vi "SMR_LabVIEW_V8.3.vi"() -> ()   [LabVIEW 2025]
uses:
  <vilib>/DAQmx/write.llb/DAQmx Write (Analog DBL 1Chan 1Samp).vi
  <vilib>/DAQmx/read.llb/DAQmx Read (Analog 1D DBL NChan 1Samp).vi
  <vilib>/DAQmx/read.llb/DAQmx Read (Analog 2D DBL NChan NSamp).vi
  <vilib>/Analysis/baseanly.llb/Mean (DBL).vi
  <vilib>/DAQmx/create/channels.llb/DAQmx Create Channel (AI-Temperature-Thermocouple).vi
  <vilib>/DAQmx/create/channels.llb/DAQmx Create Channel (AI-Voltage-Basic).vi
  <vilib>/DAQmx/create/channels.llb/DAQmx Create Channel (AO-Voltage-Basic).vi
  <vilib>/DAQmx/miscellaneous.llb/DAQmx Fill In Error Info.vi
  <vilib>/DAQmx/configure/timing.llb/DAQmx Timing (Sample Clock).vi
  <vilib>/addons/control/pid/pid.llb/PID (DBL).vi
  <vilib>/measure/maspectr.llb/FFT Power Spectrum and PSD for 1 Chan.vi
  <vilib>/measure/matone.llb/Extract Single Tone Information 1 Chan.vi
  <vilib>/addons/control/pid/NI_PID_pid.lvlib
  <vilib>/Analysis/NI_AALBase.lvlib
  <vilib>/ptbypt/NI_PtbyPt.lvlib
  <vilib>/measure/NI_MAPro.lvlib
panel:
  out "HW Valve Command (V)":dbl
  in  "HX Flow Setpoint (GPM)":dbl
  in  "Manual HW Valve Voltage (V)":dbl
  in  "HW Valve: Manual / PID":bool
  in  "PID gains for HW Valve":T1={"proportional gain (Kc)"=1.0, "integral time (Ti, min)"=0.01, "derivative time (Td, min)"=0.0} {"derivative time (Td, min)" format="%.3f"; "integral time (Ti, min)" format="%.3f"; "proportional gain (Kc)" format="%.3f"}
  out "Rod Power (W)":dbl
  out "Current Through Rod (A)":dbl
  out "Time in Steady State (s)":dbl
  in  "Steady-State Dwell (s)":dbl
  out "Main Loop Flow (GPM)":dbl
  out "FM Amplitude":dbl
  out "FM Frequency":dbl
  out "Spectrum":cluster{"f0":dbl, "df":dbl, "magnitude":dbl[]}(graph)
  out "Raw Signal":waveform(dbl)(graph)
  out "Smoothed HX Flow (GPM)":dbl
  out "Flow History":dbl(graph)
  out "HX Flow (GPM)":dbl
  out "Voltage Across Rod (V)":dbl format="%0.2f"
  out "Current Run Folder":path
  in  "Log Root Folder":path=path "C:/Users/LocalUser/Documents/GitHub/thermal-loop/resources/v0.1.1/data/001"
  out "Raw NI9201 \nVoltage Display":T2
  in  "Loop Period (ms)":dbl=1000.0
  in  "Stop":bool
  out "Auto Steady State Threshold (deg C/min)":dbl
  out "Max dT/dt (deg C/min)":dbl
  out "Temp Change Rate (deg C/min)":dbl
  out "5-Min Baseline Complete":bool
  out "Rate Window Ready":bool
  out "Steady State":bool
  in  "Voltage Limit (V)":dbl=10.0
  in  "Temperature Limit (C)":dbl=50.0
  in  "Pressure Limit (psi)":dbl=15.0
  out "Max Voltage":bool
  out "Max Temperature":bool
  out "Max Pressure":bool
  out "Heat Exchanger Pressure History":dbl(graph)
  out "Main Loop Pressure History":T3(graph)
  out "Overall Avg Pressure (psi)":dbl
  out "Heat Exchanger Pressure P6 (psi)":dbl
  out "Main Loop Avg Pressure (psi)":dbl
  out "Pressure Display":T4
  out "Overall Pressure History":T5(graph)
  out "Max Loop Pressure (psi)":dbl
  out "Heat Exchanger Temperature History":cluster{"Waveform":dbl, "Waveform":dbl}(graph)
  out "Main Loop Temeperature History":T6(graph)
  out "Heat Exchanger Avg Temp (deg C)":dbl
  out "Temperature Display":T7
  out "Overall Temperature History":T8(graph)
  out "Overall Avg Temp (deg C)":dbl
  out "Max Loop Temp (deg C)":dbl
  out "Final P-Valve Voltage (V)":dbl
  out "PID Trim Voltage (V)":dbl
  in  "PID Temp Setpoint (deg C)":dbl
  in  "Auto PID Enable":bool
  in  "Manual P-Valve Voltage (V)":dbl min=0.0 max=10.0
  out "Main Loop Avg Temp (deg C)":dbl
  # "HoneyWell Valve Control"
  # "Heat Exchanger Flow"
  # "Control/Troubleshoot"
  # "Steady State"
  # "Emergency Indicators"
  # "Pressure"
  # "Temperature"
  # "Proportional Valve Control"
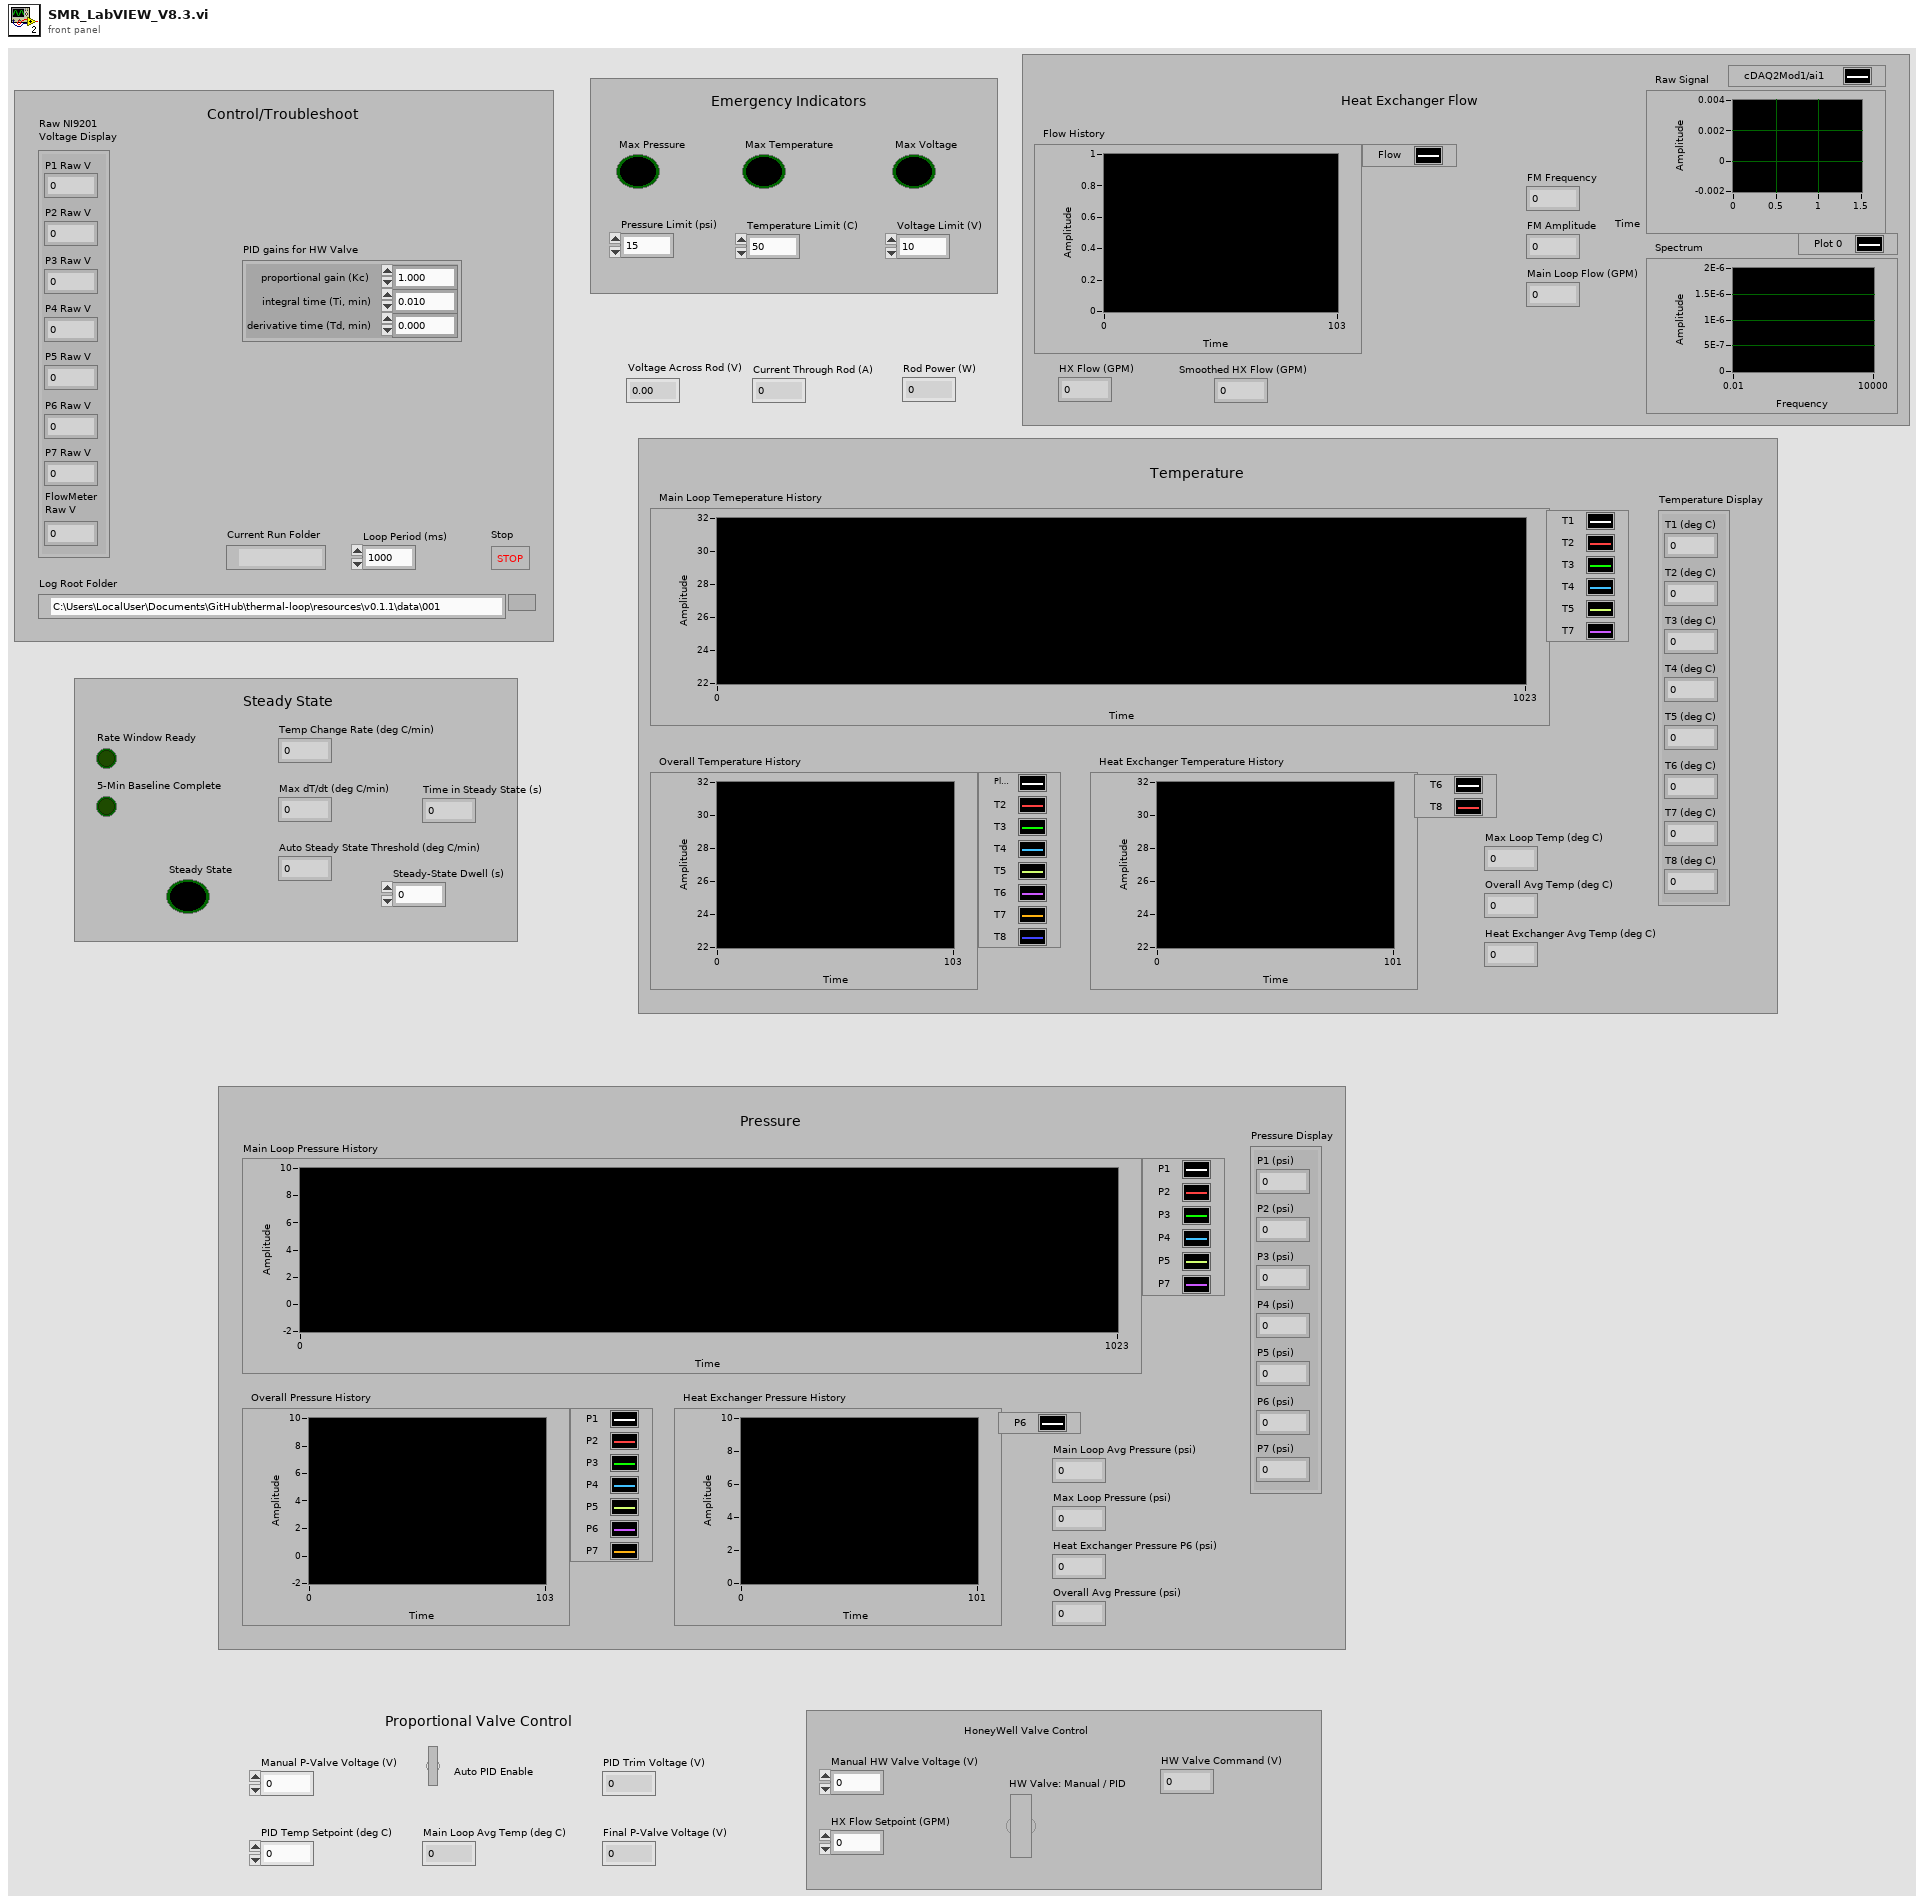
[diagram p1: front panel]
types:
  T1 = cluster{"proportional gain (Kc)":dbl, "integral time (Ti, min)":dbl, "derivative time (Td, min)":dbl}
  T2 = cluster{"P1 Raw V":dbl, "P2 Raw V":dbl, "P3 Raw V":dbl, "P4 Raw V":dbl, "P5 Raw V":dbl, "P6 Raw V":dbl, "P7 Raw V":dbl, "FlowMeter\nRaw V":dbl}
  T3 = cluster{"P1":dbl, "P2":dbl, "P3":dbl, "P4":dbl, "P5":dbl, "P7":dbl}
  T4 = cluster{"P1 (psi)":dbl, "P2 (psi)":dbl, "P3 (psi)":dbl, "P4 (psi)":dbl, "P5 (psi)":dbl, "P6 (psi)":dbl, "P7 (psi)":dbl}
  T5 = cluster{"P1":dbl, "P2":dbl, "P3":dbl, "P4":dbl, "P5":dbl, "P6":dbl, "P7":dbl}
  T6 = cluster{"Waveform":dbl, "Waveform":dbl, "Waveform":dbl, "Waveform":dbl, "Waveform":dbl, "Waveform":dbl}
  T7 = cluster{"T1 (deg C)":dbl, "T2 (deg C)":dbl, "T3 (deg C)":dbl, "T4 (deg C)":dbl, "T5 (deg C)":dbl, "T6 (deg C)":dbl, "T7 (deg C)":dbl, "T8 (deg C)":dbl}
  T8 = cluster{"Waveform":dbl, "Waveform":dbl, "Waveform":dbl, "Waveform":dbl, "Waveform":dbl, "Waveform":dbl, "Waveform":dbl, "Waveform":dbl}
  T9 = enum16{"open", "replace", "create", "open or create", "replace or create", "replace or create with confirmation"}
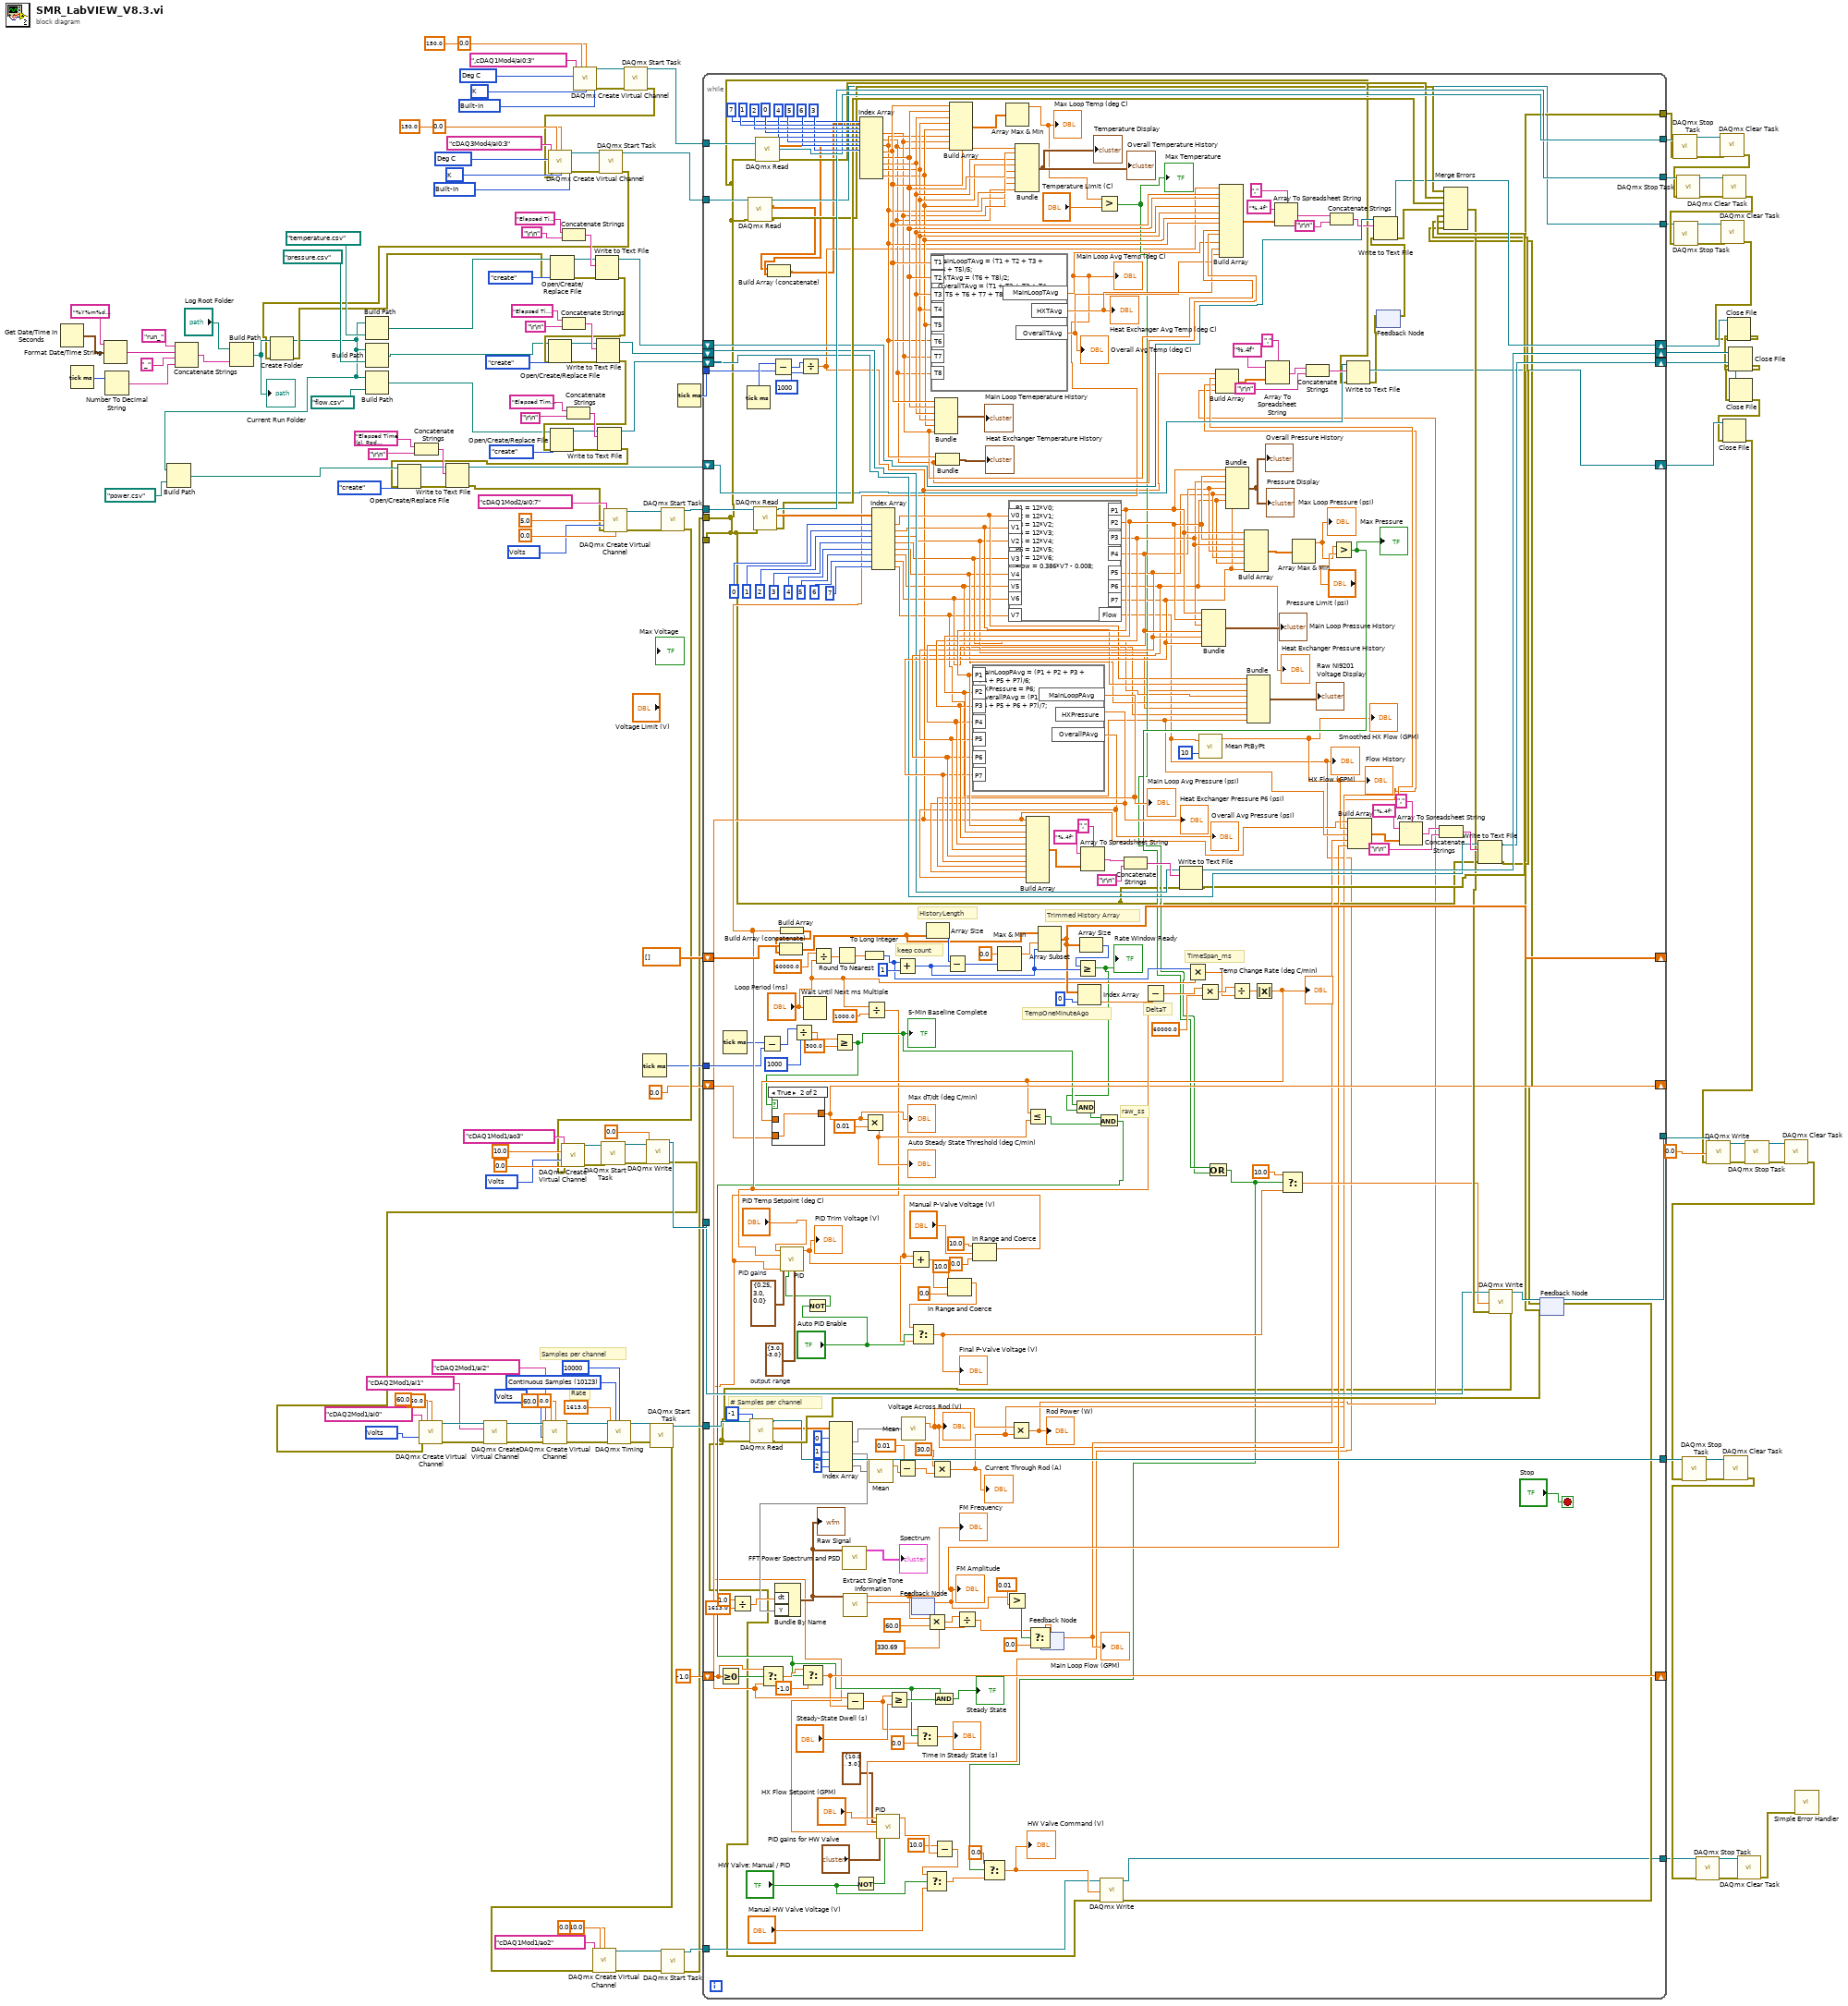
[diagram p0: block diagram]
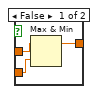
[diagram p2: hidden frame]
diagram:
  w17 = 10348 items=["Volts"=10348, "From Custom Scale"=10065] ("units")
  w34 = 10200 items=["Built-In"=10200, "Constant Value"=10116, "Channel"=10113] ("cjc source")
  w35 = 10073 items=["J"=10072, "K"=10073, "N"=10077, "R"=10082, "S"=10085, "T"=10086, "B"=10047, "E"=10055] ("thermocouple type")
  w36 = 10143 items=["Deg C"=10143, "Deg F"=10144, "Kelvins"=10325, "Deg R"=10145, "From Custom Scale"=10065] ("units")
  w66 = 10123 items=["Finite Samples"=10178, "Continuous Samples"=10123, "Hardware Timed Single Point"=12522] ("sample mode")
  w68 = 10348 items=["Volts"=10348, "From Custom Scale"=10065] ("units")
  w87 = 10348 items=["Volts"=10348, "From Custom Scale"=10065] ("units")
  w149 = 10200 items=["Built-In"=10200, "Constant Value"=10116, "Channel"=10113] ("cjc source")
  w150 = 10073 items=["J"=10072, "K"=10073, "N"=10077, "R"=10082, "S"=10085, "T"=10086, "B"=10047, "E"=10055] ("thermocouple type")
  w151 = 10143 items=["Deg C"=10143, "Deg F"=10144, "Kelvins"=10325, "Deg R"=10145, "From Custom Scale"=10065] ("units")
  w158 = 10348 items=["Volts"=10348, "From Custom Scale"=10065] ("units")
  # "Samples per channel"
  # "Rate"
  n1 = Get Date/Time In Seconds() -> (seconds since 1Jan1904=w108:timestamp)
  n2 = Tick Count (ms)() -> (millisecond timer value=w106:u32)
  n3 = Format Date/Time String(time format string (%c)="%Y%m%d_%H%M%S", seconds (now)=w108) -> (date/time string=w103:string)  [unwired: 1 in]
  n4 = Number To Decimal String(number=w106) -> (decimal integer string=w104:string)  [unwired: 1 in]
  n5 = Concatenate Strings("run_" ("string"), w103, "_" ("string"), w104) -> (w100:string)
  n6 = Build Path(base path="Log Root Folder", name or relative path=w100) -> (appended path=w99:path)
  "Current Run Folder" <- w99
  n7 = Concatenate Strings("Elapsed Time (s), Rod voltage (V), Rod Current (A), Rod Power (W)", "\r\n") -> (w53:string)
  n8 = Concatenate Strings("Elapsed Time (s),T1 (deg C),T2 (deg C),T3 (deg C),T4 (deg C),T5 (deg C),T6 (deg C),T7 (deg C),T8 (deg C),Main Loop Avg Temp (deg C),HX Avg Temp (deg C),Overall Avg Temp (deg C)", "\r\n") -> (w132:string)
  n9 = Concatenate Strings("Elapsed Time (s),P1 (psi),P2 (psi),P3 (psi),P4 (psi),P5 (psi),P6 (psi),P7 (psi),Main Loop Avg Pressure (psi),HX Pressure (psi),Overall Avg Pressure (psi)", "\r\n") -> (w130:string)
  n10 = Concatenate Strings("Elapsed Time (s),Heat Exchanger Flow (GPM),Flow Raw Voltage (V), Main Loop Flow (GPM), Flow Signal Amplitude (V)", "\r\n") -> (w126:string)
  n11 = call-poly <vilib>:"DAQmx Create Virtual Channel.vi"("maximum value"=150.0, "minimum value"=0.0, "physical channels"=tag ",cDAQ1Mod4/ai0:3", "cjc source"=w149, "units"=w151, "thermocouple type"=w150) -> ("task out"=w148:refnum<k21>, "error out"=w147:errorcluster)  [unwired: 8 in]
  n12 = call <vilib>:"DAQmx Start Task.vi"("task/channels in"=w148, "error in"=w147) -> ("task out"=w146:refnum<k21>, "error out"=w30:errorcluster)  [unwired: 12 in]
  n13 = call-poly <vilib>:"DAQmx Create Virtual Channel.vi"("maximum value"=150.0, "minimum value"=0.0, "physical channels"=tag "cDAQ3Mod4/ai0:3", "cjc source"=w34, "units"=w36, "error in"=w30, "thermocouple type"=w35) -> ("task out"=w33:refnum<k21>, "error out"=w32:errorcluster)  [unwired: 7 in]
  n14 = call <vilib>:"DAQmx Start Task.vi"("task/channels in"=w33, "error in"=w32) -> ("task out"=w28:refnum<k21>, "error out"=w29:errorcluster)  [unwired: 12 in]
  n15 = Create Folder(path (use dialog)=w99, error in=w29) -> (created path=w47:path, error out=w92:errorcluster)  [unwired: 1 in, 1 out]
  n16 = Build Path(base path=w47, name or relative path=path "power.csv") -> (appended path=w48:path)
  n17 = Build Path(base path=w47, name or relative path=path "temperature.csv") -> (appended path=w98:path)
  n18 = Build Path(base path=w47, name or relative path=path "pressure.csv") -> (appended path=w97:path)
  n19 = Build Path(base path=w47, name or relative path=path "flow.csv") -> (appended path=w96:path)
  n20 = Open/Create/Replace File(file path (use dialog)=w98, error in=w92, operation (0:open)=T9."create") -> (refnum out=w131:refnum<file>, error out=w115:errorcluster)  [unwired: 3 in, 1 out]
  n21 = Write to Text File(file (use dialog)=w131, text=w132, error in=w115) -> (refnum out=w122:refnum<file>, error out=w114:errorcluster)  [unwired: 1 in, 1 out]
  n22 = Open/Create/Replace File(file path (use dialog)=w97, error in=w114, operation (0:open)=T9."create") -> (refnum out=w129:refnum<file>, error out=w113:errorcluster)  [unwired: 3 in, 1 out]
  n23 = Write to Text File(file (use dialog)=w129, text=w130, error in=w113) -> (refnum out=w121:refnum<file>, error out=w112:errorcluster)  [unwired: 1 in, 1 out]
  n24 = Open/Create/Replace File(file path (use dialog)=w96, error in=w112, operation (0:open)=T9."create") -> (refnum out=w125:refnum<file>, error out=w111:errorcluster)  [unwired: 3 in, 1 out]
  n25 = Write to Text File(file (use dialog)=w125, text=w126, error in=w111) -> (refnum out=w120:refnum<file>, error out=w45:errorcluster)  [unwired: 1 in, 1 out]
  n26 = Open/Create/Replace File(file path (use dialog)=w48, error in=w45, operation (0:open)=T9."create") -> (refnum out=w52:refnum<file>, error out=w49:errorcluster)  [unwired: 3 in, 1 out]
  n27 = Write to Text File(file (use dialog)=w52, text=w53, error in=w49) -> (refnum out=w43:refnum<file>, error out=w44:errorcluster)  [unwired: 1 in, 1 out]
  n28 = call-poly <vilib>:"DAQmx Create Virtual Channel.vi"("maximum value"=5.0, "minimum value"=0.0, "physical channels"=tag "cDAQ1Mod2/ai0:7", "units"=w158, "error in"=w44) -> ("task out"=w157:refnum<k21>, "error out"=w156:errorcluster)  [unwired: 9 in]
  n29 = Tick Count (ms)() -> (millisecond timer value=w73:u32)
  n30 = call <vilib>:"DAQmx Start Task.vi"("task/channels in"=w157, "error in"=w156) -> ("task out"=w155:refnum<k21>, "error out"=w80:errorcluster)  [unwired: 12 in]
  n31 = call-poly <vilib>:"DAQmx Create Virtual Channel.vi"("maximum value"=10.0, "minimum value"=0.0, "physical channels"=tag "cDAQ1Mod1/ao3", "units"=w87, "error in"=w80) -> ("task out"=w86:refnum<k21>, "error out"=w85:errorcluster)  [unwired: 9 in]
  n32 = call <vilib>:"DAQmx Start Task.vi"("task/channels in"=w86, "error in"=w85) -> ("task out"=w84:refnum<k21>, "error out"=w83:errorcluster)  [unwired: 12 in]
  n33 = call-poly <vilib>:"DAQmx Write.vi"("task/channels in"=w84, "data"=0.0, "error in"=w83) -> ("task out"=w81:refnum<k21>, "error out"=w60:errorcluster)  [unwired: 10 in, 1 out]
  n34 = call-poly <vilib>:"DAQmx Create Virtual Channel.vi"("maximum value"=60.0, "minimum value"=-60.0, "physical channels"=tag "cDAQ2Mod1/ai0", "units"=w68, "error in"=w60) -> ("task out"=w57:refnum<k21>, "error out"=w56:errorcluster)  [unwired: 9 in]
  n35 = call-poly <vilib>:"DAQmx Create Virtual Channel.vi"("task in"=w57, "physical channels"=tag "cDAQ2Mod1/ai1", "error in"=w56) -> ("task out"=w21:refnum<k21>, "error out"=w19:errorcluster)  [unwired: 11 in]
  n36 = call-poly <vilib>:"DAQmx Create Virtual Channel.vi"("task in"=w21, "maximum value"=60.0, "minimum value"=-60.0, "physical channels"=tag "cDAQ2Mod1/ai2", "units"=w17, "error in"=w19) -> ("task out"=w20:refnum<k21>, "error out"=w18:errorcluster)  [unwired: 8 in]
  n37 = call-poly <vilib>:"DAQmx Timing.vi"("task/channels in"=w20, "sample mode"=w66, "samples per channel"=10000, "rate"=1613.0, "error in"=w18) -> ("task out"=w64:refnum<k21>, "error out"=w63:errorcluster)  [unwired: 9 in]
  n38 = call <vilib>:"DAQmx Start Task.vi"("task/channels in"=w64, "error in"=w63) -> ("task out"=w59:refnum<k21>, "error out"=w8:errorcluster)  [unwired: 12 in]
  n39 = call-poly <vilib>:"DAQmx Create Virtual Channel.vi"("maximum value"=10.0, "minimum value"=0.0, "physical channels"=tag "cDAQ1Mod1/ao2", "error in"=w8) -> ("task out"=w11:refnum<k21>, "error out"=w10:errorcluster)  [unwired: 10 in]
  n40 = call <vilib>:"DAQmx Start Task.vi"("task/channels in"=w11, "error in"=w10) -> ("task out"=w9:refnum<k21>, "error out"=w7:errorcluster)  [unwired: 12 in]
  n41 = Tick Count (ms)() -> (millisecond timer value=w119:u32)
  n42 = while {
    tunnel: w155 -> [w403]
    tunnel: w146 -> [w386]
    tunnel: [w377] -> w145
    tunnel: [w196] -> _
    tunnel: [w376] -> w144
    tunnel: [w255] -> w143
    shift-right: [w353] -> w118
    shift-left: w122 -> [w354]
    shift-right: [w334] -> w117
    shift-left: w121 -> [w335]
    shift-right: [w326] -> w116
    shift-left: w120 -> [w327]
    tunnel: w119 -> [w372]
    shift-right: [w305] -> _
    shift-left: dbl[] [] -> [w318]
    tunnel: w81 -> [w287]
    tunnel: w7 -> [w196]
    tunnel: [w293] -> w78
    tunnel: w73 -> [w276]
    shift-right: [w269] -> _
    shift-left: 0.0 -> [w271]
    tunnel: w59 -> [w254]
    tunnel: [w253] -> w58
    shift-right: [w213] -> w42
    shift-left: w43 -> [w214]
    shift-right: [w205] -> _
    shift-left: -1.0 -> [w209]
    tunnel: w28 -> [w197]
    tunnel: [w194] -> w24
    tunnel: w9 -> [w167]
    tunnel: [w163] -> w2
    stop <- "Stop" stop-if-true
    w291 = cluster{"output high":dbl, "output low":dbl} {"output high"=3.0, "output low"=-3.0}  # output range
    w292 = T1 {"proportional gain (Kc)"=0.25, "integral time (Ti, min)"=3.0, "derivative time (Td, min)"=0.0}  # PID gains
    # "raw_ss"
    # "# Samples per channel"
    # "TimeSpan_ms"
    # "DeltaT"
    # "TempOneMinuteAgo"
    # "Trimmed History Array"
    # "HistoryLength"
    # "keep count"
    n43 = Greater Or Equal To 0?(x=w209) -> (x >= 0?=w210:bool)
    n44 = Tick Count (ms)() -> (millisecond timer value=w277:u32)
    n45 = Divide(x=1.0, y=1613.0) -> (x/y=w227:dbl)
    n46 = Tick Count (ms)() -> (millisecond timer value=w373:u32)
    n47 = call-poly <vilib>:"DAQmx Read.vi"("task/channels in"=w197, "error in"=w196) -> ("task out"=w194:refnum<k21>, "data"=w191:dbl[], "error out"=w195:errorcluster)  [unwired: 11 in]
    n48 = call-poly <vilib>:"DAQmx Read.vi"("task/channels in"=w403, "error in"=w196) -> ("task out"=w376:refnum<k21>, "data"=w394:dbl[], "error out"=w374:errorcluster)  [unwired: 11 in]
    n49 = call-poly <vilib>:"DAQmx Read.vi"("task/channels in"=w386, "error in"=w196) -> ("task out"=w377:refnum<k21>, "data"=w192:dbl[], "error out"=w375:errorcluster)  [unwired: 11 in]
    n50 = Subtract(x=w277, y=w276) -> (x-y=w275:u32)
    n51 = Build Array (concatenate)(w191, w192) -> (w193:dbl[])
    n52 = Subtract(x=w373, y=w372) -> (x-y=w371:u32)
    n53 = Divide(x=w275, y=u32 1000) -> (x/y=w273:dbl)
    n54 = Divide(x=w371, y=u32 1000) -> (x/y=w206:dbl)
    n55 = Select(t=w209, s=w210, f=w206) -> (s? t:f=w208:dbl)
    n56 = Wait Until Next ms Multiple(millisecond multiple="Loop Period (ms)") -> ()  [unwired: 1 out]
    n57 = Not(x="Auto PID Enable") -> (.not. x?=w288:bool)
    n58 = Divide(x=60000.0, y="Loop Period (ms)") -> (x/y=w315:dbl)
    n59 = Greater Or Equal?(x=w273, y=300.0) -> (x >= y?=w266:bool)
    "5-Min Baseline Complete" <- w266
    n60 = Round To Nearest(number=w315) -> (nearest integer value=w314:dbl)
    n61 = Not(x="HW Valve: Manual / PID") -> (.not. x?=w177:bool)
    n62 = Index Array(array=w193, index #1=7 ("index"), index #2=1 ("index"), index #3=2 ("index"), index #4=0 ("index"), index #5=4 ("index"), index #6=5 ("index"), index #7=6 ("index"), index #8=3 ("index")) -> (element #1=w363:dbl, element #2=w362:dbl, element #3=w364:dbl, element #4=w369:dbl, element #5=w368:dbl, element #6=w367:dbl, element #7=w366:dbl, element #8=w365:dbl)
    n63 = To Long Integer(number=w314) -> (32bit integer=w302:i32)
    n64 = Divide(x="Loop Period (ms)", y=1000.0) -> (x/y=w162:dbl)
    n65 = Index Array(array=w394, index #1=0 ("index"), index #2=1 ("index"), index #3=2 ("index"), index #4=3 ("index"), index #5=4 ("index"), index #6=5 ("index"), index #7=6 ("index"), index #8=7 ("index")) -> (element #1=w252:dbl, element #2=w251:dbl, element #3=w250:dbl, element #4=w249:dbl, element #5=w248:dbl, element #6=w247:dbl, element #7=w246:dbl, element #8=w245:dbl)
    n66 = Add(x=w302, y=1) -> (x+y=w307:i32)
    n67 = feedback #1() -> (w223:dbl)  [unwired: 1 in]
    "FM Amplitude" <- w223
    n68 = formula code="MainLoopTAvg = (T1 + T2 + T3 + T4 + T5)/5;\nHXTAvg = (T6 + T8)/2;\nOverallTAvg = (T1 + T2 + T3 + T4 + T5 + T6 + T7 + T8)/8;"("T1"=w369, "T2"=w368, "T3"=w367, "T4"=w366, "T5"=w365, "T6"=w364, "T7"=w363, "T8"=w362) -> ("MainLoopTAvg"=w279:dbl, "HXTAvg"=w361:dbl, "OverallTAvg"=w360:dbl)
    "Overall Avg Temp (deg C)" <- w360
    "Main Loop Avg Temp (deg C)" <- w279
    "Heat Exchanger Avg Temp (deg C)" <- w361
    n69 = Build Array(w279) -> (w317:dbl[])
    n70 = Build Array (concatenate)(w318, w317) -> (w309:dbl[])
    n71 = call-poly <vilib>:"PID.vi"("reinitialize? (F)"=w288, "output range"=w291, "dt (s)"=w162, "PID gains"=w292, "process variable"=w279, "setpoint"="PID Temp Setpoint (deg C)") -> ("output"=w286:dbl)  [unwired: 4 in, 1 out]
    "PID Trim Voltage (V)" <- w286
    n72 = Array Size(array=w309) -> (size(s)=w312:i32)
    n73 = Bundle("Waveform"=w369, "Waveform"=w368, "Waveform"=w367, "Waveform"=w366, "Waveform"=w365, "Waveform"=w363) -> (→"Main Loop Temeperature History":T6)  [unwired: 1 in]
    n74 = Bundle("Waveform"=w364, "Waveform"=w362) -> (→"Heat Exchanger Temperature History":cluster{"Waveform":dbl, "Waveform":dbl})  [unwired: 1 in]
    n75 = Subtract(x=w312, y=w307) -> (x-y=w310:i32)
    n76 = Build Array(w369, w368, w367, w366, w365, w364, w363, w362) -> (w404:dbl[])
    n77 = In Range and Coerce(upper limit=10.0, x="Manual P-Valve Voltage (V)", lower limit=0.0) -> (coerced(x)=w281:dbl)  [unwired: 1 out]
    n78 = Add(x=w281, y=w286) -> (x+y=w285:dbl)
    n79 = In Range and Coerce(upper limit=10.0, x=w285, lower limit=0.0) -> (coerced(x)=w280:dbl)  [unwired: 1 out]
    n80 = Select(t=w280, s="Auto PID Enable", f=w281) -> (s? t:f=w258:dbl)
    "Final P-Valve Voltage (V)" <- w258
    n81 = Max & Min(x=0.0, y=w310) -> (max(x,y)=w308:dbl)  [unwired: 1 out]
    n82 = Array Max & Min(array=w404) -> (max value=w320:dbl)  [unwired: 3 out]
    "Max Loop Temp (deg C)" <- w320
    n83 = Greater?(x=w223, y=0.01) -> (0:w231:bool)
    n84 = formula code="P1 = 12*V0;\nP2 = 12*V1;\nP3 = 12*V2;\nP4 = 12*V3;\nP5 = 12*V4;\nP6 = 12*V5; \nP7 = 12*V6;\nFlow = 0.386*V7 - 0.008;"("V0"=w252, "V1"=w251, "V2"=w250, "V3"=w249, "V4"=w248, "V5"=w247, "V6"=w246, "V7"=w245) -> ("P1"=w352:dbl, "P2"=w351:dbl, "P3"=w350:dbl, "P4"=w349:dbl, "P5"=w348:dbl, "P6"=w347:dbl, "P7"=w346:dbl, "Flow"=w180:dbl)
    "HX Flow (GPM)" <- w180
    "Heat Exchanger Pressure History" <- w347
    n85 = call-poly <vilib>:"PID.vi"("reinitialize? (F)"=w177, "output range"=cluster{"output high":dbl, "output low":dbl} {"output high"=10.0, "output low"=3.0}, "dt (s)"=w162, "PID gains"="PID gains for HW Valve", "process variable"=w180, "setpoint"="HX Flow Setpoint (GPM)") -> ("output"=w176:dbl)  [unwired: 4 in, 1 out]
    n86 = Subtract(x=10.0, y=w176) -> (x-y=w173:dbl)
    n87 = Select(t=w173, s="HW Valve: Manual / PID", f="Manual HW Valve Voltage (V)") -> (s? t:f=w170:dbl)
    n88 = formula code="MainLoopPAvg = (P1 + P2 + P3 + P4 + P5 + P7)/6;\nHXPressure = P6;\nOverallPAvg = (P1 + P2 + P3 + P4 + P5 + P6 + P7)/7;"("P1"=w352, "P2"=w351, "P3"=w350, "P4"=w349, "P5"=w348, "P6"=w347, "P7"=w346) -> ("MainLoopPAvg"=w345:dbl, "HXPressure"=w344:dbl, "OverallPAvg"=w343:dbl)
    "Overall Avg Pressure (psi)" <- w343
    "Heat Exchanger Pressure P6 (psi)" <- w344
    "Main Loop Avg Pressure (psi)" <- w345
    n89 = Bundle("Waveform"=w369, "Waveform"=w368, "Waveform"=w367, "Waveform"=w366, "Waveform"=w365, "Waveform"=w364, "Waveform"=w363, "Waveform"=w362) -> (→"Overall Temperature History" →"Temperature Display":T8)  [unwired: 1 in]
    n90 = Build Array(w206, w352, w351, w350, w349, w348, w347, w346, w345, w344, w343) -> (w342:dbl[])
    n91 = Array Subset(array=w309, index=w308, length=w307) -> (w305:dbl[])
    n92 = feedback #2() -> (w221:dbl)  [unwired: 1 in]
    "Main Loop Flow (GPM)" <- w221
    n93 = Index Array(array=w305, index=0) -> (element=w303:dbl)
    n94 = Array Size(array=w305) -> (size(s)=w306:i32)
    n95 = Greater Or Equal?(x=w306, y=w307) -> (x >= y?=w265:bool)
    "Rate Window Ready" <- w265
    n96 = And(x=w266, y=w265) -> (x .and. y?=w264:bool)
    n97 = Array To Spreadsheet String(delimiter (Tab)=",", array=w342, 3:"%.4f" ("format string")) -> (spreadsheet string=w338:string)
    n98 = Greater?(x=w320, y="Temperature Limit (C)") -> (0:w261:bool)
    "Max Temperature" <- w261
    n99 = Concatenate Strings(w338, "\r\n") -> (w336:string)
    n100 = Subtract(x=w279, y=w303) -> (x-y=w301:dbl)
    n101 = Write to Text File(file (use dialog)=w335, text=w336, error in=w196) -> (refnum out=w334:refnum<file>, error out=w324:errorcluster)  [unwired: 1 in, 1 out]
    n102 = Multiply(x=w302, y="Loop Period (ms)") -> (x*y=w298:dbl)
    n103 = Multiply(x=w301, y=60000.0) -> (x*y=w299:dbl)
    n104 = call <vilib>:"Mean PtByPt.vi"("x"=w180, "sample length"=10) -> ("mean"=w243:dbl)  [unwired: 2 in, 1 out]
    "Flow History" <- w243
    "Smoothed HX Flow (GPM)" <- w243
    n105 = Bundle("P1"=w352, "P2"=w351, "P3"=w350, "P4"=w349, "P5"=w348, "P7"=w346) -> (→"Main Loop Pressure History":T3)  [unwired: 1 in]
    n106 = Build Array(w206, w369, w368, w367, w366, w365, w364, w363, w362, w279, w361, w360) -> (w359:dbl[])
    n107 = Bundle("P1"=w352, "P2"=w351, "P3"=w350, "P4"=w349, "P5"=w348, "P6"=w347, "P7"=w346) -> (→"Overall Pressure History" →"Pressure Display":T5)  [unwired: 1 in]
    n108 = Divide(x=w299, y=w298) -> (x/y=w297:dbl)
    n109 = Build Array(w352, w351, w350, w349, w348, w347, w346) -> (w393:dbl[])
    n110 = Bundle("Waveform"=w252, "Waveform"=w251, "Waveform"=w250, "Waveform"=w249, "Waveform"=w248, "Waveform"=w247, "Waveform"=w246, "Waveform"=w245) -> (→"Raw NI9201 \nVoltage Display":T8)  [unwired: 1 in]
    n111 = Absolute Value(x=w297) -> (abs(x)=w268:dbl)
    "Temp Change Rate (deg C/min)" <- w268
    n112 = case shown="True" w266 {
      tunnel: w271 -> [w408 w409]
      tunnel: w268 -> [w407 _]
      tunnel: [w406 w409] -> w269
      frame False {
        n113 = Max & Min(x=w407, y=w408) -> (max(x,y)=w406:dbl)  [unwired: 1 out]
      }
      frame True {
      }
    }
    "Max dT/dt (deg C/min)" <- w269
    n114 = Multiply(x=w269, y=0.01) -> (x*y=w267:dbl)
    "Auto Steady State Threshold (deg C/min)" <- w267
    n115 = Less Or Equal?(x=w268, y=w267) -> (x <= y?=w263:bool)
    n116 = And(x=w264, y=w263) -> (x .and. y?=w201:bool)
    n117 = Select(t=w208, s=w201, f=-1.0) -> (s? t:f=w205:dbl)
    n118 = Subtract(x=w206, y=w205) -> (x-y=w200:dbl)
    n119 = Greater Or Equal?(x=w200, y="Steady-State Dwell (s)") -> (x >= y?=w203:bool)
    n120 = Select(t=w200, s=w201, f=0.0) -> (s? t:f=→"Time in Steady State (s)":dbl)
    n121 = And(x=w201, y=w203) -> (x .and. y?=→"Steady State":bool)
    n122 = Array To Spreadsheet String(delimiter (Tab)=",", array=w359, 3:"%.4f" ("format string")) -> (spreadsheet string=w356:string)
    n123 = Array Max & Min(array=w393) -> (max value=w321:dbl)  [unwired: 3 out]
    "Max Loop Pressure (psi)" <- w321
    n124 = Concatenate Strings(w356, "\r\n") -> (w339:string)
    n125 = Greater?(x=w321, y="Pressure Limit (psi)") -> (0:w262:bool)
    "Max Pressure" <- w262
    n126 = Or(x=w262, y=w261) -> (x .or. y?=w171:bool)
    n127 = Select(t=0.0, s=w171, f=w170) -> (s? t:f=w168:dbl)
    "HW Valve Command (V)" <- w168
    n128 = Select(t=10.0, s=w171, f=w258) -> (s? t:f=w257:dbl)
    n129 = Build Array(w206, w243, w245, w221, w223) -> (w333:dbl[])
    n130 = feedback #3() -> (w211:errorcluster)  [unwired: 1 in]
    n131 = Write to Text File(file (use dialog)=w354, text=w339, error in=w211) -> (refnum out=w353:refnum<file>, error out=w325:errorcluster)  [unwired: 1 in, 1 out]
    n132 = Array To Spreadsheet String(delimiter (Tab)=",", array=w333, 3:"%.4f" ("format string")) -> (spreadsheet string=w329:string)
    n133 = Concatenate Strings(w329, "\r\n") -> (w328:string)
    n134 = Write to Text File(file (use dialog)=w327, text=w328, error in=w196) -> (refnum out=w326:refnum<file>, error out=w323:errorcluster)  [unwired: 1 in, 1 out]
    n135 = feedback #4() -> (w164:errorcluster)  [unwired: 1 in]
    n136 = Merge Errors(w195, w375, w374, w325, w324, w323, w164) -> (w294:errorcluster)
    n137 = call-poly <vilib>:"DAQmx Write.vi"("task/channels in"=w287, "data"=w257, "error in"=w294) -> ("task out"=w293:refnum<k21>, "error out"=w166:errorcluster)  [unwired: 10 in, 1 out]
    n138 = call-poly <vilib>:"DAQmx Read.vi"("task/channels in"=w254, "number of samples per channel"=-1, "error in"=w166) -> ("task out"=w253:refnum<k21>, "data"=w242:dbl[][], "error out"=w255:errorcluster)  [unwired: 10 in]
    n139 = Index Array(array=w242, index (row) #1=0 ("index (row)"), index (row) #2=1 ("index (row)"), index (row) #3=2 ("index (row)")) -> (element #1=w241:dbl[], element #2=w226:dbl[], element #3=w186:dbl[])  [unwired: 3 in]
    n140 = Bundle By Name("dt"=w227, "Y"=w226) -> (w225:waveform(dbl))  [unwired: 1 in]
    "Raw Signal" <- w225
    n141 = call-poly <vilib>:"FFT Power Spectrum and PSD.vi"("time signal"=w225) -> ("Power Spectrum / PSD"=→"Spectrum":cluster{"f0":dbl, "df":dbl, "magnitude":dbl[]})  [unwired: 7 in, 3 out]
    n142 = call-poly <vilib>:"Extract Single Tone Information.vi"("time signal in"=w225) -> ("detected amplitude"=w224:dbl, "detected frequency"=w237:dbl)  [unwired: 5 in, 4 out]
    "FM Frequency" <- w237
    n143 = call-poly <vilib>:"Mean.vi"("X"=w186) -> ("mean"=w187:dbl)  [unwired: 1 out]
    n144 = Subtract(x=0.01, y=w187) -> (x-y=w188:dbl)
    n145 = call-poly <vilib>:"Mean.vi"("X"=w241) -> ("mean"=w184:dbl)  [unwired: 1 out]
    "Voltage Across Rod (V)" <- w184
    n146 = feedback-in #1(w224) -> ()
    n147 = Multiply(x=w237, y=60.0) -> (x*y=w235:dbl)
    n148 = Multiply(x=30.0, y=w188) -> (x*y=w183:dbl)
    "Current Through Rod (A)" <- w183
    n149 = Divide(x=w235, y=330.69) -> (x/y=w230:dbl)
    n150 = Multiply(x=w184, y=w183) -> (x*y=w182:dbl)
    "Rod Power (W)" <- w182
    n151 = Select(t=w230, s=w231, f=0.0) -> (s? t:f=w222:dbl)
    n152 = feedback-in #2(w222) -> ()
    n153 = call-poly <vilib>:"DAQmx Write.vi"("task/channels in"=w167, "data"=w168, "error in"=w166) -> ("task out"=w163:refnum<k21>, "error out"=w165:errorcluster)  [unwired: 10 in, 1 out]
    n154 = Build Array(w206, w184, w183, w182) -> (w216:dbl[])
    n155 = Array To Spreadsheet String(delimiter (Tab)=",", array=w216, 3:"%.4f" ("format string")) -> (spreadsheet string=w219:string)
    n156 = Concatenate Strings(w219, "\r\n") -> (w215:string)
    n157 = Write to Text File(file (use dialog)=w214, text=w215, error in=w196) -> (refnum out=w213:refnum<file>, error out=w212:errorcluster)  [unwired: 1 in, 1 out]
    n158 = feedback-in #3(w212) -> ()
    n159 = feedback-in #4(w165) -> ()
  }
  n160 = call <vilib>:"DAQmx Stop Task.vi"("task/channels in"=w145, "error in"=w143) -> ("task out"=w142:refnum<k21>, "error out"=w140:errorcluster)  [unwired: 12 in]
  n161 = call <vilib>:"DAQmx Clear Task.vi"("task in"=w142, "error in"=w140) -> ("error out"=w139:errorcluster)  [unwired: 13 in]
  n162 = call <vilib>:"DAQmx Stop Task.vi"("task/channels in"=w144, "error in"=w139) -> ("task out"=w141:refnum<k21>, "error out"=w138:errorcluster)  [unwired: 12 in]
  n163 = call <vilib>:"DAQmx Clear Task.vi"("task in"=w141, "error in"=w138) -> ("error out"=w27:errorcluster)  [unwired: 13 in]
  n164 = call <vilib>:"DAQmx Stop Task.vi"("task/channels in"=w24, "error in"=w27) -> ("task out"=w23:refnum<k21>, "error out"=w26:errorcluster)  [unwired: 12 in]
  n165 = call <vilib>:"DAQmx Clear Task.vi"("task in"=w23, "error in"=w26) -> ("error out"=w25:errorcluster)  [unwired: 13 in]
  n166 = Close File(refnum=w118, error in=w25) -> (error out=w110:errorcluster)  [unwired: 1 out]
  n167 = Close File(refnum=w117, error in=w110) -> (error out=w109:errorcluster)  [unwired: 1 out]
  n168 = Close File(refnum=w116, error in=w109) -> (error out=w41:errorcluster)  [unwired: 1 out]
  n169 = Close File(refnum=w42, error in=w41) -> (error out=w40:errorcluster)  [unwired: 1 out]
  n170 = call-poly <vilib>:"DAQmx Write.vi"("task/channels in"=w78, "data"=0.0, "error in"=w40) -> ("task out"=w77:refnum<k21>, "error out"=w75:errorcluster)  [unwired: 10 in, 1 out]
  n171 = call <vilib>:"DAQmx Stop Task.vi"("task/channels in"=w77, "error in"=w75) -> ("task out"=w76:refnum<k21>, "error out"=w74:errorcluster)  [unwired: 12 in]
  n172 = call <vilib>:"DAQmx Clear Task.vi"("task in"=w76, "error in"=w74) -> ("error out"=w6:errorcluster)  [unwired: 13 in]
  n173 = call <vilib>:"DAQmx Stop Task.vi"("task/channels in"=w58, "error in"=w6) -> ("task out"=w62:refnum<k21>, "error out"=w61:errorcluster)  [unwired: 12 in]
  n174 = call <vilib>:"DAQmx Clear Task.vi"("task in"=w62, "error in"=w61) -> ("error out"=w3:errorcluster)  [unwired: 13 in]
  n175 = call <vilib>:"DAQmx Stop Task.vi"("task/channels in"=w2, "error in"=w3) -> ("task out"=w5:refnum<k21>, "error out"=w4:errorcluster)  [unwired: 12 in]
  n176 = call <vilib>:"DAQmx Clear Task.vi"("task in"=w5, "error in"=w4) -> ("error out"=w1:errorcluster)  [unwired: 13 in]
  n177 = call <vilib>:"Simple Error Handler.vi"("error in (no error)"=w1) -> ()  [unwired: 4 in, 5 out]
